vi "DAQmx_set_AI_autorange.vi"(8 "error in (no error)":errorcluster, 9 "multiplier":dbl=1.0 min=1.0, 11 "task/channels in":refnum<k21>) -> (0 "error out":errorcluster, 3 "task out":refnum<k21>, 4 "AI.Max":dbl, 6 "AI.Min":dbl)   [LabVIEW 2017]
uses:
  <vilib>/DAQmx/read.llb/DAQmx Read (Analog DBL 1Chan 1Samp).vi
  <vilib>/DAQmx/miscellaneous.llb/DAQmx Fill In Error Info.vi
  <resource>/objmgr/daqmx.rc
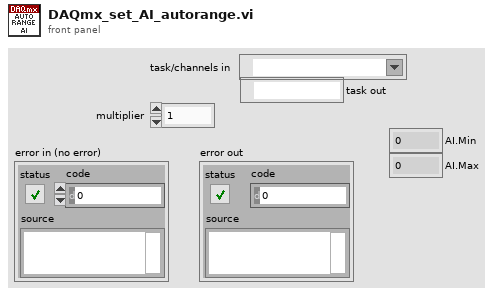
[diagram p1: front panel]
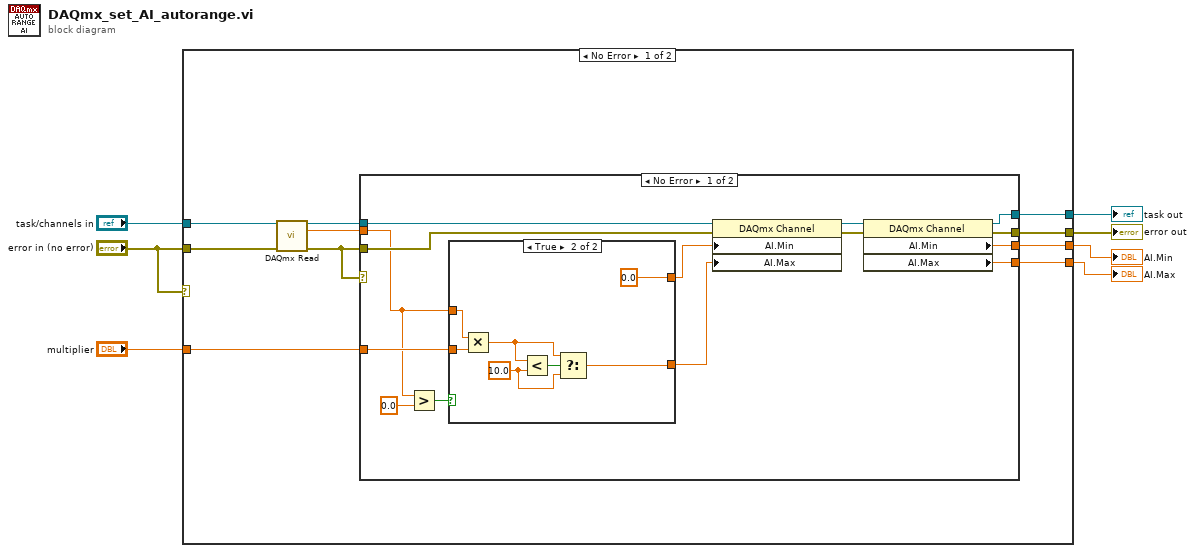
[diagram p0: block diagram]
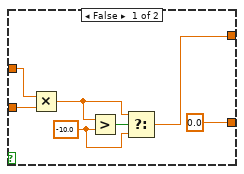
[diagram p2: hidden frame]
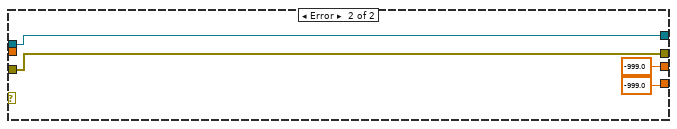
[diagram p3: hidden frame]
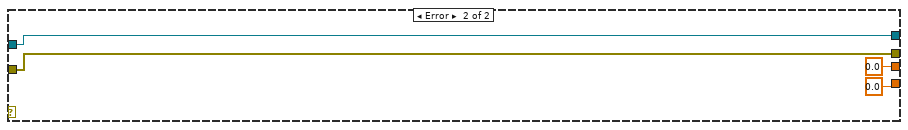
[diagram p4: hidden frame]
diagram:
  n1 = case shown="No Error" "error in (no error)" {
    tunnel: [w12 w52] -> w7
    tunnel: "error in (no error)" -> [w16 w52]
    tunnel: "task/channels in" -> [w15 w53]
    tunnel: [w13 w53] -> w5
    tunnel: "multiplier" -> [w14 _]
    tunnel: [w11 0.0 ("AI.Min")] -> w2
    tunnel: [w10 0.0 ("AI.Max")] -> w1
    frame No Error {
      n2 = call-poly <vilib>:"DAQmx Read.vi"("task/channels in"=w15, "error in"=w16) -> ("task out"=w17:refnum<k21>, "data"=w9:dbl, "error out"=w8:errorcluster)  [unwired: 11 in]
      n3 = case shown="No Error" w8 {
        tunnel: w17 -> [w31 w49]
        tunnel: w8 -> [w30 w48]
        tunnel: w14 -> [w29 _]
        tunnel: [w26 w49] -> w13
        tunnel: [w25 w48] -> w12
        tunnel: [w24 -999.0 ("AI.Min")] -> w11
        tunnel: [w23 -999.0 ("AI.Max")] -> w10
        tunnel: w9 -> [w20 _]
        frame No Error {
          n4 = Greater?(x=w20, y=0.0) -> (0:w22:bool)
          n5 = case shown="True" w22 {
            tunnel: w20 -> [w34 w41]
            tunnel: [w32 0.0 ("AI.Min")] -> w19
            tunnel: w29 -> [w35 w42]
            tunnel: [0.0 ("AI.Min") w39] -> w18
            frame False {
              w36 = -10.0 ("y")
              n6 = Multiply(x=w34, y=w35) -> (x*y=w38:dbl)
              n7 = Greater?(x=w38, y=w36) -> (0:w37:bool)
              n8 = Select(t=w38, s=w37, f=w36) -> (s? t:f=w32:dbl)
            }
            frame True {
              w40 = 10.0 ("y")
              n9 = Multiply(x=w41, y=w42) -> (x*y=w44:dbl)
              n10 = Less?(x=w44, y=w40) -> (x < y?=w43:bool)
              n11 = Select(t=w44, s=w43, f=w40) -> (s? t:f=w39:dbl)
            }
          }
          n12 = property class="DAQmx Channel"(reference=w31, error in=w30, "AI.Min"=w19, "AI.Max"=w18) -> (reference out=w27:refnum<k21>, error out=w28:errorcluster)
          n13 = property class="DAQmx Channel"(reference=w27, error in=w28) -> (reference out=w26:refnum<k21>, error out=w25:errorcluster, "AI.Min"=w24:dbl, "AI.Max"=w23:dbl)
        }
        frame Error {
        }
      }
    }
    frame Error {
    }
  }
  "error out" <- w7
  "task out" <- w5
  "AI.Min" <- w2
  "AI.Max" <- w1
